vi "Check if Custom Device Enabled.vi"(8 "error in":errorcluster, 11 "custom device ref in":T1 format="%.0x") -> (0 "error out":errorcluster, 2 "Custom Device is Enabled":bool, 3 "custom device ref out":T1 format="%.0x")   [LabVIEW 2020, in "Communication Bus Template Scripting.lvlib"]
uses:
  Communication Bus Template Scripting.lvlib
  <vilib>/NI VeriStand/Custom Device API/Custom Device Item Ref.ctl
  Constants.vi
  <vilib>/NI VeriStand/Custom Device API/Custom Device API.lvlib
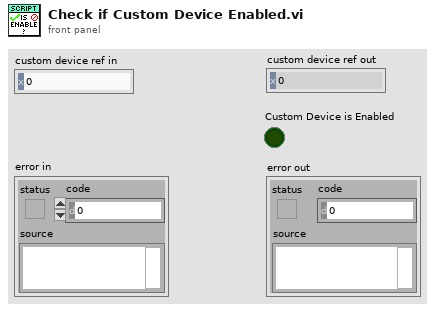
[diagram p1: front panel]
types:
  T1 = typedef "Custom Device API.lvlib/Custom Device Item Ref.ctl" = u64
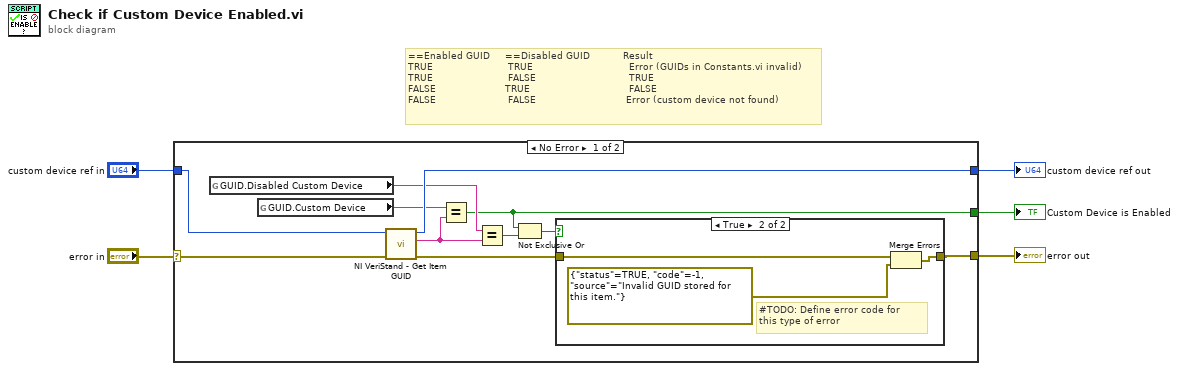
[diagram p0: block diagram]
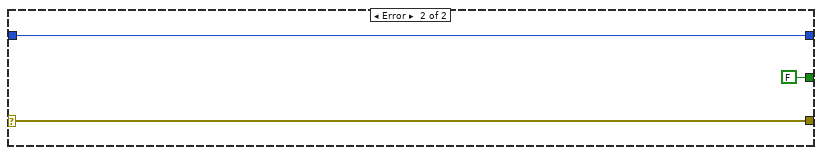
[diagram p3: hidden frame]
diagram:
  # "==Enabled GUID     ==Disabled GUID           Result\nTRUE                         TRUE                                Error (GUIDs in Constants.vi invalid)\nTRUE                         FALSE                               TRUE\nFALSE                       TRUE                                 FALSE\nFALSE                        FALSE                              Error (custom device not found)"
  n1 = case shown="No Error" "error in" {
    selector: "error in" -> [w16 w23]
    tunnel: [w14 w23] -> w4
    tunnel: [w12 w22] -> w3
    tunnel: "custom device ref in" -> [w13 w22]
    tunnel: [w6 FALSE] -> w1
    frame No Error {
      n2 = global read "Constants.vi" "GUID.Disabled Custom Device"() -> (w10:string)
      n3 = global read "Constants.vi" "GUID.Custom Device"() -> (w11:string)
      n4 = call <vilib>:"NI VeriStand - Get Item GUID.vi"("error in (no error)"=w16, "Item Ref in"=w13) -> ("error out"=w15:errorcluster, "GUID"=w9:string, "Item Ref out"=w12:T1)  [unwired: 7 in]
      n5 = Equal?(x=w11, y=w9) -> (x = y?=w6:bool)
      n6 = Equal?(x=w10, y=w9) -> (x = y?=w7:bool)
      n7 = Not Exclusive Or(1:w7, 2:w6) -> (0:w8:bool)
      n8 = case shown="True" w8 {
        tunnel: [w17 w19] -> w14
        tunnel: w15 -> [w17 w18]
        frame False {
        }
        frame True {
          # "#TODO: Define error code for\nthis type of error"
          n9 = Merge Errors(w18, errorcluster {"status"=TRUE, "code"=-1, "source"="Invalid GUID stored for this item."} ("New Error")) -> (w19:errorcluster)
        }
      }
    }
    frame Error {
    }
  }
  "custom device ref out" <- w3
  "error out" <- w4
  "Custom Device is Enabled" <- w1
